vi "VI Tree.vi"   [LabVIEW 2012, in "Agilent 66XX Series.lvlib"]
doc: "Displays all the VI of the instrument driver in an organized table."
uses:
  <instrlib>/Agilent 66XX Series/Agilent 66XX Series.lvlib
panel:
  # "© 2005 National Instruments.  ALL RIGHTS RESERVED."
  # "See Diagram Box\nfor VI Tree"
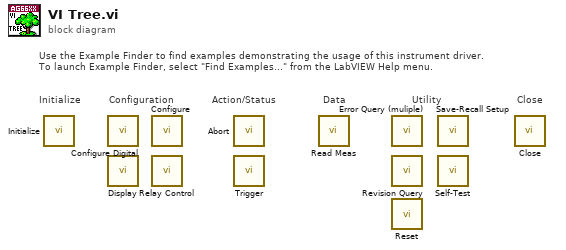
[diagram p0: block diagram]
diagram:
  # "Use the Example Finder to find examples demonstrating the usage of this instrument driver.\nTo launch Example Finder, select \"Find Examples...\" from the LabVIEW Help menu."
  # "Close"
  # "Utility"
  # "Data"
  # "Action/Status"
  # "Configuration"
  # "Initialize"
  n1 = call <instrlib>:"Initialize.vi"() -> ()  [unwired: 14 in, 2 out]
  n2 = call <instrlib>:"Configure Digital.vi"() -> ()  [unwired: 14 in, 2 out]
  n3 = call <instrlib>:"Display.vi"() -> ()  [unwired: 14 in, 2 out]
  n4 = call <instrlib>:"Configure.vi"() -> ()  [unwired: 14 in, 2 out]
  n5 = call <instrlib>:"Relay Control.vi"() -> ()  [unwired: 14 in, 2 out]
  n6 = call <instrlib>:"Abort.vi"() -> ()  [unwired: 14 in, 2 out]
  n7 = call <instrlib>:"Trigger.vi"() -> ()  [unwired: 14 in, 2 out]
  n8 = call <instrlib>:"Read Meas.vi"() -> ()  [unwired: 12 in, 4 out]
  n9 = call <instrlib>:"Error Query (muliple).vi"() -> ()  [unwired: 12 in, 4 out]
  n10 = call <instrlib>:"Revision Query.vi"() -> ()  [unwired: 12 in, 4 out]
  n11 = call <instrlib>:"Reset.vi"() -> ()  [unwired: 14 in, 2 out]
  n12 = call <instrlib>:"Save-Recall Setup.vi"() -> ()  [unwired: 14 in, 2 out]
  n13 = call <instrlib>:"Self-Test.vi"() -> ()  [unwired: 12 in, 4 out]
  n14 = call <instrlib>:"Close.vi"() -> ()  [unwired: 15 in, 1 out]
